vi "Get all Object Items.vi"(8 "error in (no error)":errorcluster, 10 "Offset":i32, 11 "JSON":string) -> (0 "error out":errorcluster, 1 "<JSON>":string[](array[string]) caption="<JSON>Items", 2 "Offset past":i32 caption="Offset past Object", 3 "Item Names":string[](array[string]))   [LabVIEW 2024, in "JSONtext.lvlib"]
doc: "Return all Items in the Object as an array of JSON Values."
uses:
  JSONtext.lvlib
  Advance past whitespace.vi
  Advance past whitespace and comma.vi
  Advance past colon.vi
  Advance past String.vi
  Advance past next JSON Scaler.vi
  String Subset.vi
  Strip Quotes and Unescape.vi
  Advance past Line Ending.vi
  Advance past Number.vi
  Unescape JSON string.vi
  Advance past Object.vi
  Advance past Array.vi
  Parsing Error.vi
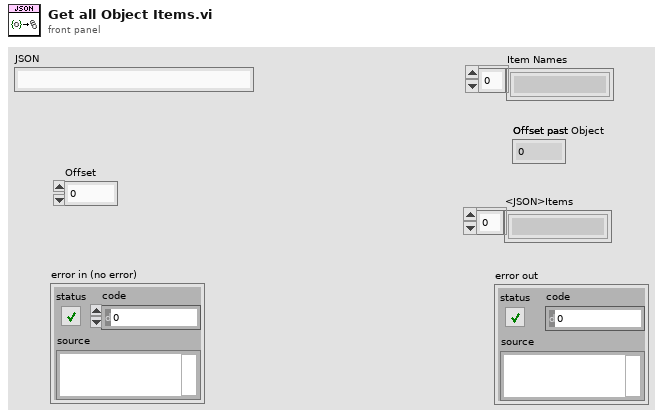
[diagram p1: front panel]
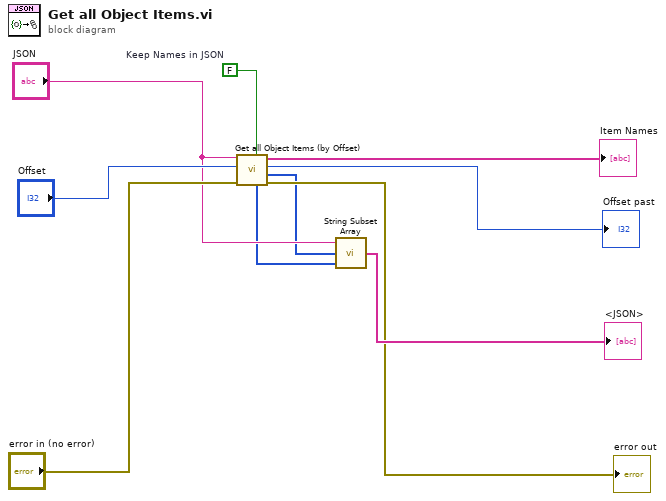
[diagram p0: block diagram]
diagram:
  w1 = FALSE  # Keep Names in JSON
  n1 = call "Get all Object Items (by Offset).vi"("Keep Names in JSON"=w1, "error in (no error)"="error in (no error)", "Offset"="Offset", "JSON"="JSON") -> ("error out"=→"error out":errorcluster, "Item Offsets"=w3:i32[], "Offset past"=→"Offset past":i32, "Item Names"=→"Item Names":string[], "Item End Offsets"=w2:i32[])  [unwired: 3 in]
  n2 = call "String Subset Array.vi"("Offset past End"=w2, "Start offset"=w3, "JSON"="JSON") -> ("Subsets"=→"<JSON>":string[])  [unwired: 2 in]
